vi "Conversion_between_Cluster_Types-1.vi"(1 "[IN] New Movie Values":T2 {"Particle Fil Setups"."Type of particle filter"."Measurement Parameter" items=["Center of Mass X", "Center of Mass Y", "First Pixel X", "First Pixel Y", "Bounding Rect Left", "Bounding Rect Top", "Bounding Rect Right", "Bounding Rect Bottom", "Max Feret Diameter Start X", "Max Feret Diameter Start Y", "Max Feret Diameter End X", "Max Feret Diameter End Y", "Max Horiz. Segment Length Left", "Max Horiz. Segment Length Right", "Max Horiz. Segment Length Row", "-", "Bounding Rect Width", "Bounding Rect Height", "Bounding Rect Diagonal", "Perimeter", "Convex Hull Perimeter", "Holes' Perimeter", "Max Feret Diameter", "Equivalent Ellipse Major Axis", "Equivalent Ellipse Minor Axis", "Equivalent Ellipse Minor Axis (Feret)", "Equivalent Rect Long Side", "Equivalent Rect Short Side", "Equivalent Rect Diagonal", "Equivalent Rect Short Side (Feret)", "Average Horiz. Segment Length", "Average Vert. Segment Length", "Hydraulic Radius", "Waddel Disk Diameter", "-", "Area", "Holes' Area", "Particle & Holes' Area", "Convex Hull Area", "Image Area", "-", "Number of Holes", "Number of Horiz. Segments", "Number of Vert. Segments", "-", "Orientation", "Max Feret Diameter Orientation", "-", "% Area/Image Area", "% Area/(Particle & Holes' Area)", "Ratio of Equivalent Ellipse Axes", "Ratio of Equivalent Rect Sides", "-", "Elongation Factor", "Compactness Factor", "Heywood Circularity Factor", "Type Factor", "-", "Sum X", "Sum Y", "Sum XX", "Sum XY", "Sum YY", "Sum XXX", "Sum XXY", "Sum XYY", "Sum YYY", "-", "Moment of Inertia XX", "Moment of Inertia XY", "Moment of Inertia YY", "Moment of Inertia XXX", "Moment of Inertia XXY", "Moment of Inertia XYY", "Moment of Inertia YYY", "Norm. Moment of Inertia XX", "Norm. Moment of Inertia XY", "Norm. Moment of Inertia YY", "Norm. Moment of Inertia XXX", "Norm. Moment of Inertia XXY", "Norm. Moment of Inertia XYY", "Norm. Moment of Inertia YYY", "Hu Moment 1", "Hu Moment 2", "Hu Moment 3", "Hu Moment 4", "Hu Moment 5", "Hu Moment 6", "Hu Moment 7"]}) -> (0 "[OUT] Old Movie Values":T3 {"Particle Fil Setups"."Type of particle filter"."Measurement Parameter" items=["Center of Mass X", "Center of Mass Y", "First Pixel X", "First Pixel Y", "Bounding Rect Left", "Bounding Rect Top", "Bounding Rect Right", "Bounding Rect Bottom", "Max Feret Diameter Start X", "Max Feret Diameter Start Y", "Max Feret Diameter End X", "Max Feret Diameter End Y", "Max Horiz. Segment Length Left", "Max Horiz. Segment Length Right", "Max Horiz. Segment Length Row", "-", "Bounding Rect Width", "Bounding Rect Height", "Bounding Rect Diagonal", "Perimeter", "Convex Hull Perimeter", "Holes' Perimeter", "Max Feret Diameter", "Equivalent Ellipse Major Axis", "Equivalent Ellipse Minor Axis", "Equivalent Ellipse Minor Axis (Feret)", "Equivalent Rect Long Side", "Equivalent Rect Short Side", "Equivalent Rect Diagonal", "Equivalent Rect Short Side (Feret)", "Average Horiz. Segment Length", "Average Vert. Segment Length", "Hydraulic Radius", "Waddel Disk Diameter", "-", "Area", "Holes' Area", "Particle & Holes' Area", "Convex Hull Area", "Image Area", "-", "Number of Holes", "Number of Horiz. Segments", "Number of Vert. Segments", "-", "Orientation", "Max Feret Diameter Orientation", "-", "% Area/Image Area", "% Area/(Particle & Holes' Area)", "Ratio of Equivalent Ellipse Axes", "Ratio of Equivalent Rect Sides", "-", "Elongation Factor", "Compactness Factor", "Heywood Circularity Factor", "Type Factor", "-", "Sum X", "Sum Y", "Sum XX", "Sum XY", "Sum YY", "Sum XXX", "Sum XXY", "Sum XYY", "Sum YYY", "-", "Moment of Inertia XX", "Moment of Inertia XY", "Moment of Inertia YY", "Moment of Inertia XXX", "Moment of Inertia XXY", "Moment of Inertia XYY", "Moment of Inertia YYY", "Norm. Moment of Inertia XX", "Norm. Moment of Inertia XY", "Norm. Moment of Inertia YY", "Norm. Moment of Inertia XXX", "Norm. Moment of Inertia XXY", "Norm. Moment of Inertia XYY", "Norm. Moment of Inertia YYY", "Hu Moment 1", "Hu Moment 2", "Hu Moment 3", "Hu Moment 4", "Hu Moment 5", "Hu Moment 6", "Hu Moment 7"]})   [LabVIEW 2013]
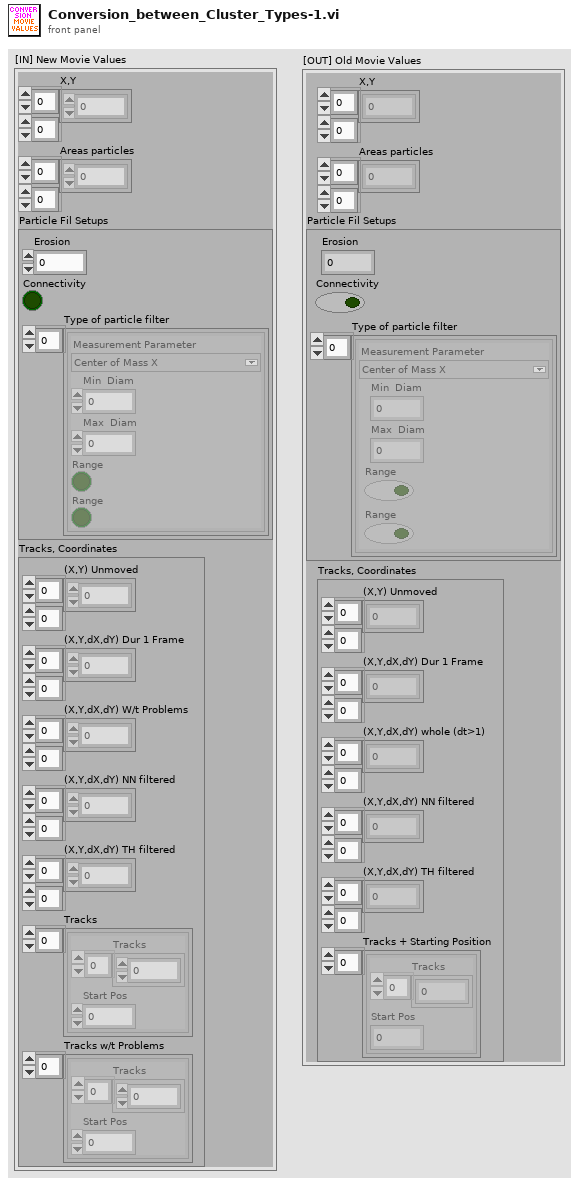
[diagram p1: front panel]
types:
  T1 = typedef "Particle Parameters" = i32
  T2 = cluster{"X,Y":dbl[][], "Areas particles":dbl[][], "Particle Fil Setups":cluster{"Erosion":i32, "Connectivity ":bool, "Type of particle filter":cluster{"Measurement Parameter":T1, "Min  Diam":dbl, "Max  Diam":dbl, "Range":bool, "Range":bool}[]}, "Tracks, Coordinates":cluster{"(X,Y) Unmoved":dbl[][], "(X,Y,dX,dY) Dur 1 Frame":dbl[][], "(X,Y,dX,dY) W/t Problems":dbl[][], "(X,Y,dX,dY) NN filtered":dbl[][], "(X,Y,dX,dY) TH filtered":dbl[][], "Tracks":cluster{"Tracks":dbl[], "Start Pos":i32}[], "Tracks w/t Problems":cluster{"Tracks":dbl[], "Start Pos":i32}[]}}
  T3 = cluster{"X,Y":dbl[][], "Areas particles":dbl[][], "Particle Fil Setups":cluster{"Erosion":i32, "Connectivity ":bool, "Type of particle filter":cluster{"Measurement Parameter":T1, "Min  Diam":dbl, "Max  Diam":dbl, "Range":bool, "Range":bool}[]}, "Tracks, Coordinates":cluster{"(X,Y) Unmoved":dbl[][], "(X,Y,dX,dY) Dur 1 Frame":dbl[][], "(X,Y,dX,dY) whole (dt>1)":dbl[][], "(X,Y,dX,dY) NN filtered":dbl[][], "(X,Y,dX,dY) TH filtered":dbl[][], "Tracks + Starting Position":cluster{"Tracks":dbl[], "Start Pos":i32}[]}}
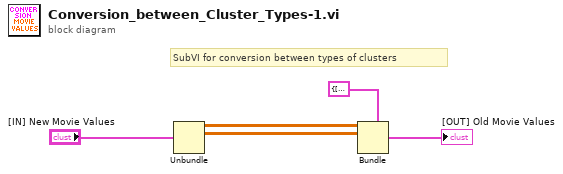
[diagram p0: block diagram]
diagram:
  # "SubVI for conversion between types of clusters"
  n1 = Unbundle("[IN] New Movie Values") -> ("X,Y"=w3:dbl[][], "Areas particles"=w2:dbl[][])  [unwired: 2 out]
  n2 = Bundle(cluster=T3 {"X,Y"=[], "Areas particles"=[], "Particle Fil Setups"={"Erosion"=0, "Connectivity "=FALSE, "Type of particle filter"=[]}, "Tracks, Coordinates"={"(X,Y) Unmoved"=[], "(X,Y,dX,dY) Dur 1 Frame"=[], "(X,Y,dX,dY) whole (dt>1)"=[], "(X,Y,dX,dY) NN filtered"=[], "(X,Y,dX,dY) TH filtered"=[], "Tracks + Starting Position"=[]}} ("[OUT] Old Movie Values"), "X,Y"=w3, "Areas particles"=w2) -> (→"[OUT] Old Movie Values":T3)  [unwired: 2 in]
